vi "estructura_casos_num.vi"() -> ()   [LabVIEW 2020]
panel:
  in  "Boolean":bool
  out "RESULTADO":dbl
  in  "Valor 2":dbl
  in  "Valor 1":dbl
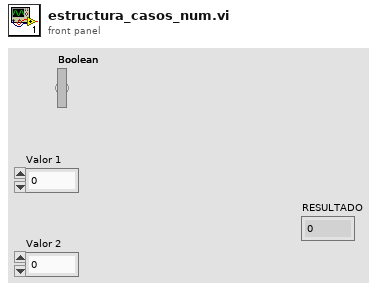
[diagram p1: front panel]
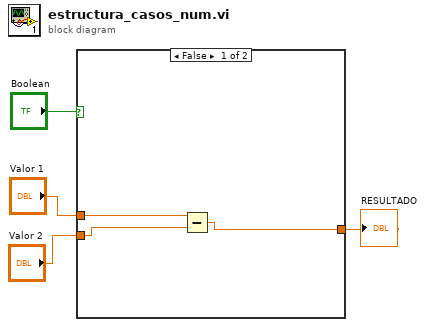
[diagram p0: block diagram]
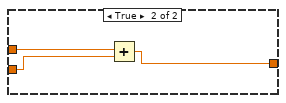
[diagram p2: hidden frame]
diagram:
  n1 = case shown="False" "Boolean" {
    tunnel: "Valor 1" -> [w7 w10]
    tunnel: "Valor 2" -> [w6 w9]
    tunnel: [w5 w8] -> w2
    frame False {
      n2 = Subtract(x=w7, y=w6) -> (x-y=w5:dbl)
    }
    frame True {
      n3 = Add(x=w10, y=w9) -> (x+y=w8:dbl)
    }
  }
  "RESULTADO" <- w2
